vi "Server_Remove User.vi"(7 "connection ID":refnum<k5>, 8 "error in":errorcluster, 11 "User Data":T1={"Name"="Guset", "Email"="", "Phone Number"="", "User Picture"=array225x225[50625 elements], "Last Login Time"=timestamp(0 s since 1904-01-01)}) -> (0 "error out":errorcluster, 3 "OK?":bool)   [LabVIEW 2018, in "Cloud Server.lvlib"]
uses:
  Cloud Server.lvlib
  Com VIs/Data Def/User Data.ctl
  Data Def/Server_Connection Manager Method.ctl
  Data Def/Server_Connection Properties.ctl
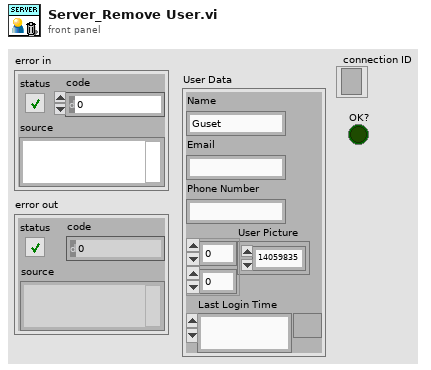
[diagram p1: front panel]
types:
  T1 = typedef "User Data.ctl" = cluster{"Name":string, "Email":string, "Phone Number":string, "User Picture":u32[][], "Last Login Time":timestamp}
  T2 = typedef "Cloud Server.lvlib/Server_Connection Properties.ctl" = cluster{"User Data":T1, "Data":waveform(dbl)}
  T3 = typedef "Cloud Server.lvlib/Server_Connection Manager Method.ctl" = enum16{"Initialize", "Add", "Get", "Set Properties", "Get Properties", "Close", "Release"}
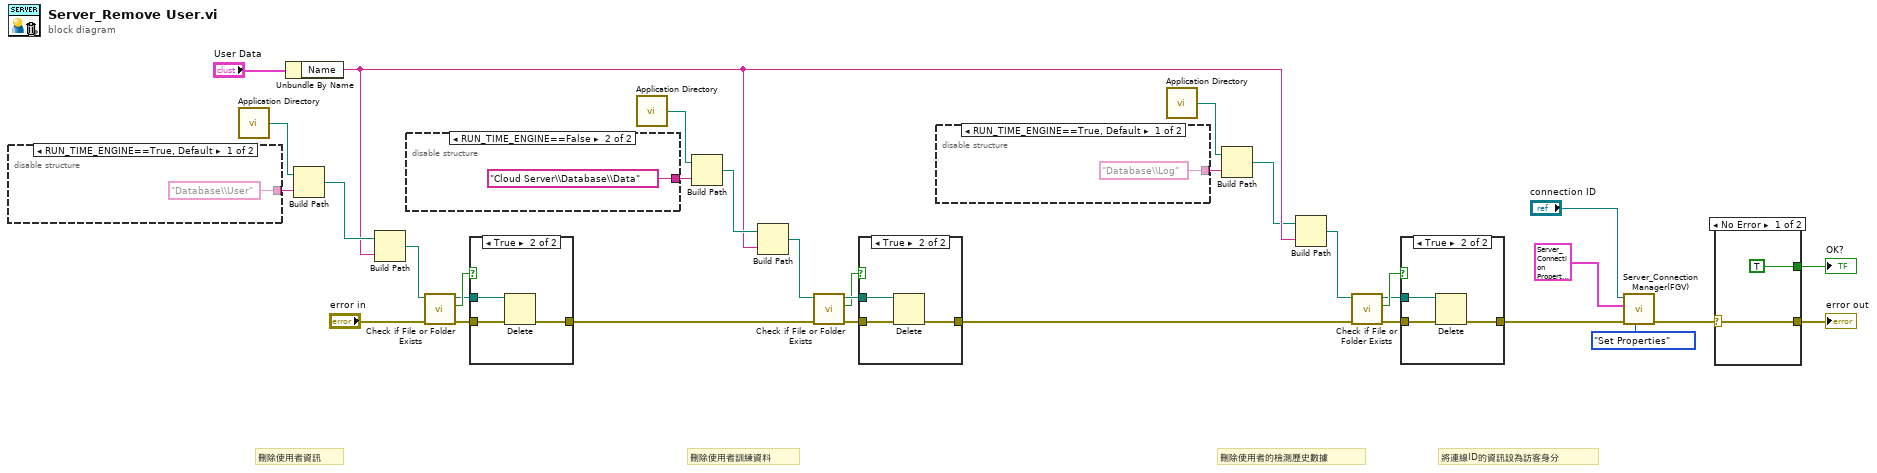
[diagram p0: block diagram]
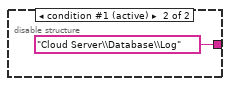
[diagram p3: hidden frame]
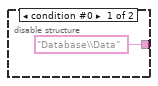
[diagram p6: hidden frame]
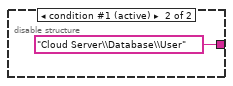
[diagram p8: hidden frame]
diagram:
  # "將連線ID的資訊設為訪客身分"
  # "刪除使用者的檢測歷史數據"
  # "刪除使用者訓練資料"
  # "刪除使用者資訊"
  n1 = disable-structure shown="RUN_TIME_ENGINE==True, Default" {
    disable-tunnel: ["Database\\User" ("name or relative path") "Cloud Server\\Database\\User" ("name or relative path")] -> w32
    frame condition #0 {
    }
    frame condition #1 (active) {
    }
  }
  n2 = call <vilib>:"Application Directory.vi"() -> ("Application Directory"=w31:path)
  n3 = Unbundle By Name("User Data") -> ("Name"=w8:string)
  n4 = Build Path(base path=w31, name or relative path=w32) -> (appended path=w30:path)
  n5 = Build Path(base path=w30, name or relative path=w8) -> (appended path=w21:path)
  n6 = disable-structure shown="RUN_TIME_ENGINE==False" {
    disable-tunnel: ["Database\\Data" ("name or relative path") "Cloud Server\\Database\\Data" ("name or relative path")] -> w23
    frame condition #0 {
    }
    frame condition #1 (active) {
    }
  }
  n7 = call <vilib>:"Check if File or Folder Exists.vi"("error in (no error)"="error in", "path"=w21) -> ("error out"=w19:errorcluster, "file or folder exists?"=w18:bool, "dup path"=w17:path)  [unwired: 7 in]
  n8 = case shown="True" w18 {
    tunnel: w19 -> [w38 w41]
    tunnel: w17 -> [_ w40]
    tunnel: [w38 w39] -> w13
    frame False {
    }
    frame True {
      n9 = Delete(path (use dialog)=w40, error in=w41) -> (error out=w39:errorcluster)  [unwired: 3 in, 2 out]
    }
  }
  n10 = call <vilib>:"Application Directory.vi"() -> ("Application Directory"=w22:path)
  n11 = Build Path(base path=w22, name or relative path=w23) -> (appended path=w12:path)
  n12 = Build Path(base path=w12, name or relative path=w8) -> (appended path=w11:path)
  n13 = call <vilib>:"Check if File or Folder Exists.vi"("error in (no error)"=w13, "path"=w11) -> ("error out"=w14:errorcluster, "file or folder exists?"=w15:bool, "dup path"=w16:path)  [unwired: 7 in]
  n14 = case shown="True" w15 {
    tunnel: w14 -> [w42 w45]
    tunnel: w16 -> [_ w44]
    tunnel: [w42 w43] -> w6
    frame False {
    }
    frame True {
      n15 = Delete(path (use dialog)=w44, error in=w45) -> (error out=w43:errorcluster)  [unwired: 3 in, 2 out]
    }
  }
  n16 = disable-structure shown="RUN_TIME_ENGINE==True, Default" {
    disable-tunnel: ["Database\\Log" ("name or relative path") "Cloud Server\\Database\\Log" ("name or relative path")] -> w9
    frame condition #0 {
    }
    frame condition #1 (active) {
    }
  }
  n17 = call <vilib>:"Application Directory.vi"() -> ("Application Directory"=w10:path)
  n18 = Build Path(base path=w10, name or relative path=w9) -> (appended path=w7:path)
  n19 = Build Path(base path=w7, name or relative path=w8) -> (appended path=w5:path)
  n20 = call <vilib>:"Check if File or Folder Exists.vi"("error in (no error)"=w6, "path"=w5) -> ("error out"=w4:errorcluster, "file or folder exists?"=w3:bool, "dup path"=w2:path)  [unwired: 7 in]
  n21 = case shown="True" w3 {
    tunnel: w4 -> [w48 w51]
    tunnel: w2 -> [_ w50]
    tunnel: [w48 w49] -> w1
    frame False {
    }
    frame True {
      n22 = Delete(path (use dialog)=w50, error in=w51) -> (error out=w49:errorcluster)  [unwired: 3 in, 2 out]
    }
  }
  n23 = call "Server_Connection Manager(FGV).vi"("Connection Manager Method(Get)"=Server_Connection_Manager_Method."Set Properties", "error in"=w1, "Connection Properties In"=T2 {"User Data"={"Name"="Guest", "Email"="", "Phone Number"="", "User Picture"=array225x225[50625 elements], "Last Login Time"=timestamp(0 s since 1904-01-01)}, "Data"={"t0"=timestamp(0 s since 1904-01-01), "dt"=1.0, "Y"=[]}}, "Connection In"="connection ID") -> ("error out"=w27:errorcluster)  [unwired: 3 in, 4 out]
  n24 = case shown="No Error" w27 {
    selector: w27 -> [w53 _]
    tunnel: [w53 _] -> w26
    tunnel: [TRUE _] -> w25
    frame No Error {
    }
    frame Error {
    }
  }
  "error out" <- w26
  "OK?" <- w25
